vi "MPS_global_variables.vi"() -> ()   [LabVIEW 2021]
panel:
  in  "Rx TF File":string="MPS_Rx_TF_10TurnCoilInput_Pos142.mat"
  in  "Fan Control Line":tag="H1/port0/line6"
  in  "mT/Bias Amp":dbl=9.36
  in  "mT/Drive Amp":dbl=0.65
  in  "Drive IMon\nRef Freq":dbl=23809.0
  in  "Volts Per Amp\nBias":dbl=0.034
  in  "Volts Per Amp\nDrive":dbl=0.008
  out "mT/BMon Volt":dbl=19.346166678499063
  in  "Analog Input Start Trig":tag="/H1/ai/StartTrigger"
  in  "Bias Output Chan.":tag="H1/ao1"
  in  "Drive Output Chan.":tag="H1/ao0"
  in  "B-Mon chan. mode":i32(ring)=10083 items=["Default"=-1, "RSE"=10083, "NRSE"=10078, "Differential"=10106, "Pseudodifferential"=12529]
  in  "Rx chan. mode":i32(ring)=10106 items=["Default"=-1, "RSE"=10083, "NRSE"=10078, "Differential"=10106, "Pseudodifferential"=12529]
  in  "B-Mon sense channel":tag="H1/ai6"
  in  "Drive I-Mon chan. mode":i32(ring)=10083 items=["Default"=-1, "RSE"=10083, "NRSE"=10078, "Differential"=10106, "Pseudodifferential"=12529]
  in  "Bias I-Mon chan. mode":i32(ring)=10083 items=["Default"=-1, "RSE"=10083, "NRSE"=10078, "Differential"=10106, "Pseudodifferential"=12529]
  in  "Rx channel":tag="H1/ai7"
  in  "Drive current meas. channel":tag="H1/ai4"
  in  "Bias I-Mon channel":tag="H1/ai5"
  in  "TxRx_Params":T1={"sample rate"=1000000.0, "Tx freq"=23809.52380952381, "Tx amp"=0.5, "Tx cycles\nSpectroscopy"=500.0, "Bias amp"=2.65, "Bias freq"=11.904761904761905, "Receive range"=5.0, "Bias Periods\nMagnetometry"=20.0, "Tx Freq Division Factor"=42.0, "Drive Periods per Bias"=2000.0, "TX harmonics"=[47619.04761904762, 71428.57142857142, 95238.09523809524, 119047.61904761905, 142857.14285714284, 166666.66666666666, 190476.19047619047, 214285.7142857143, 238095.2380952381, 261904.7619047619, 285714.2857142857, 309523.8095238095, 333333.3333333333, 357142.85714285716, 380952.38095238095, 404761.90476190473, 428571.4285714286, 452380.95238095237, 476190.4761904762, 500000.0]} {"TX harmonics" format="%#_4p"}
  in  "Device Name":tag="DAQ2"
  # "DAQ settings"
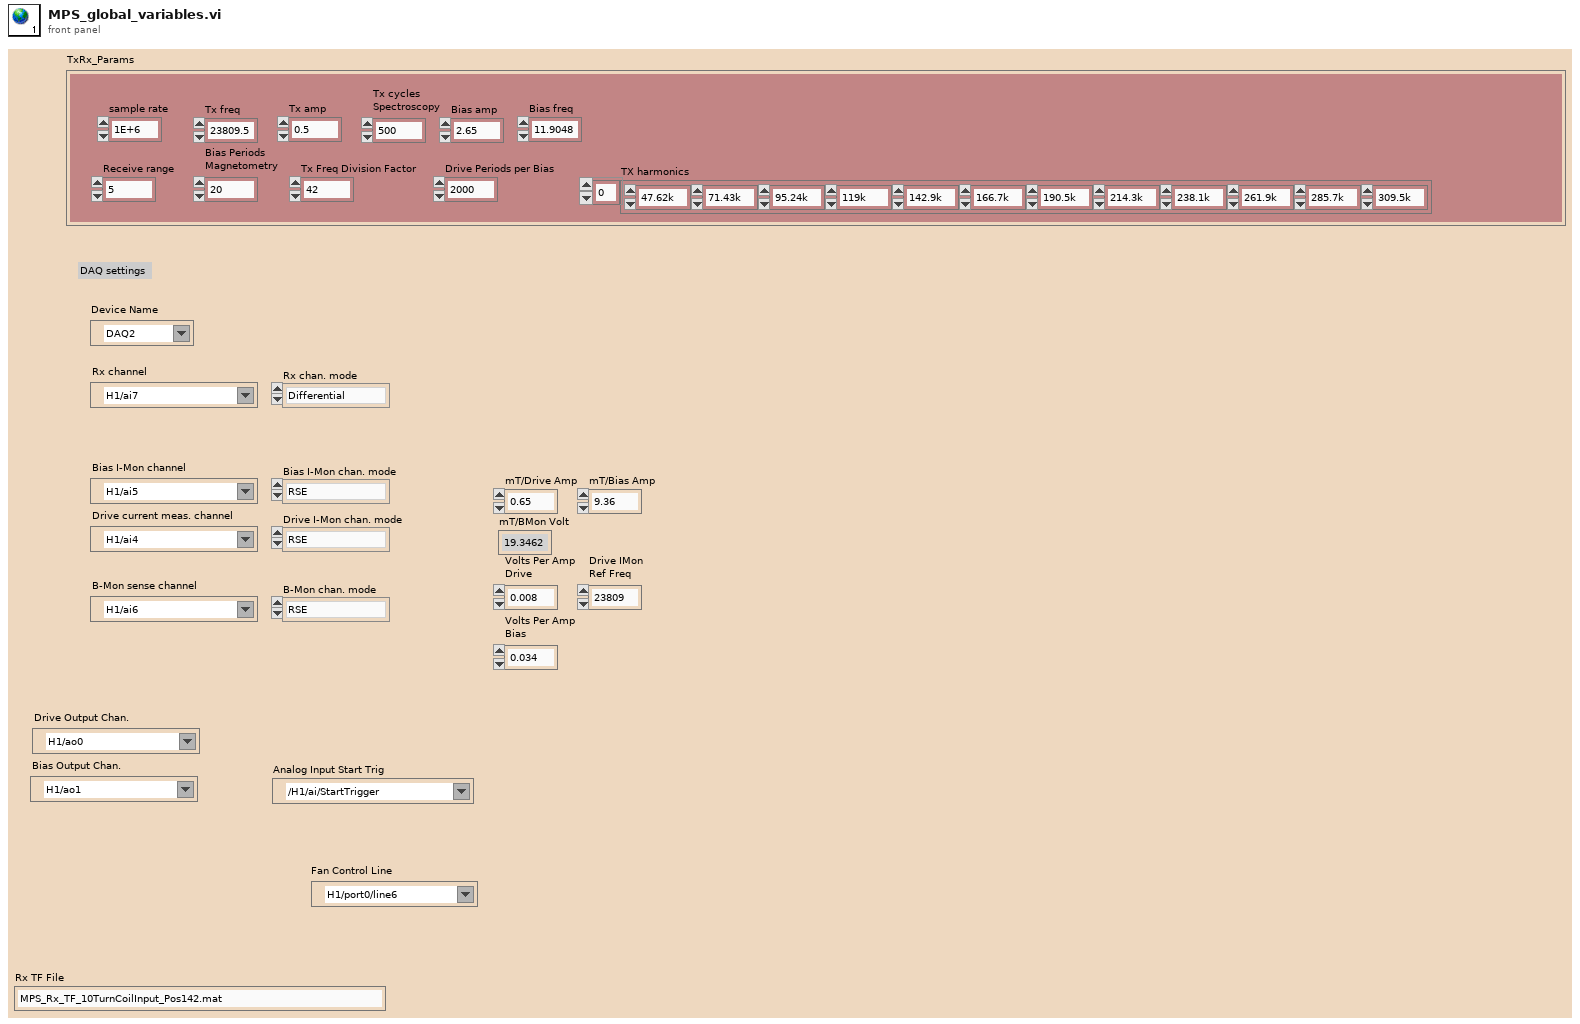
[diagram p1: front panel]
types:
  T1 = cluster{"sample rate":dbl, "Tx freq":dbl, "Tx amp":dbl, "Tx cycles\nSpectroscopy":dbl, "Bias amp":dbl, "Bias freq":dbl, "Receive range":dbl, "Bias Periods\nMagnetometry":dbl, "Tx Freq Division Factor":dbl, "Drive Periods per Bias":dbl, "TX harmonics":dbl[]}
diagram:
